vi "SummaryWithGlyphManager.vi"(8 "error in":errorcluster, 9 "glyph manager":T1, 10 "depth":i32, 11 "node self ref":T3) -> (0 "error out":errorcluster, 1 "glyph manager out":T1, 2 "summary":T4[](array[typedef]))   [LabVIEW 2025, in "CEF.lvlib"]
doc: "Gets the summary of a node and all the subnodes. This description can be used to update the tree controlCopyright 2017 National Instruments Corporation\n\nLicensed under the Apache License, Version 2.0 (the \"License\"); you may not use this file except in compliance with the License. You may obtain a copy of the License at http://www.apache.org/licenses/LICENSE-2.0\nUnless required by applicable law or agreed to in writing, software distributed under the License is distributed on an \"AS IS\" BASIS, WITHOUT WARRANTIES OR CONDITIONS OF ANY KIND, either express or implied. See the License for the specific language governing permissions and limitations under the License."
uses:
  CEF.lvlib
  Node/Summary.ctl
  Node/NodeRef.ctl
  Node/CEF_Node.lvclass
  glyph manager/glyph manager.ctl
  <vilib>/picture/picture.llb/imagedata.ctl
  Node/CEF_Node.lvclass/CEF_Node.ctl
  Node/ReadParent.vi
  Node/ReadChildren.vi
  Node/ReadNodeClass.vi
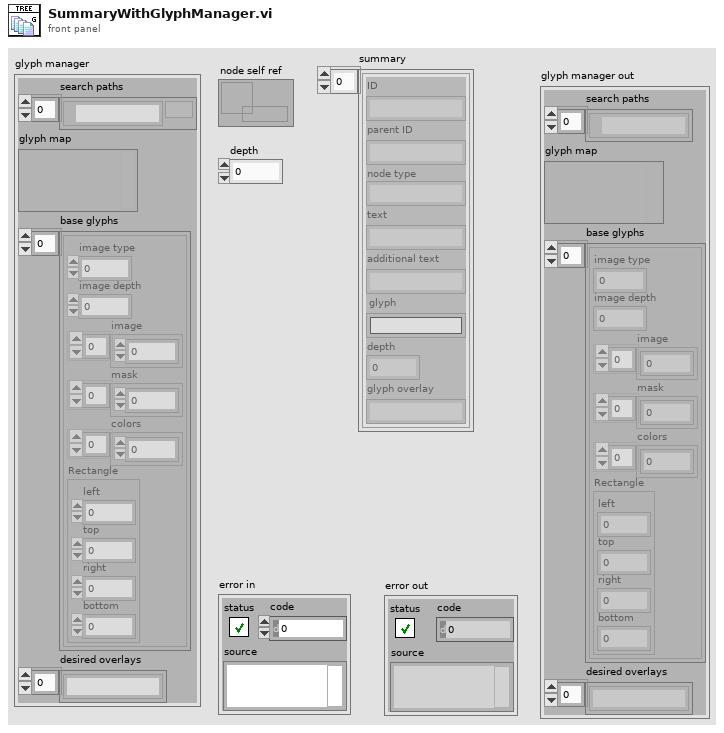
[diagram p1: front panel]
types:
  T1 = typedef "CEF.lvlib/glyph manager.ctl" = cluster{"search paths":path[], "glyph map":variant, "base glyphs":T2[], "desired overlays":string[]}
  T2 = typedef "imagedata.ctl" = cluster{"image type":i32, "image depth":i32, "image":u8[], "mask":u8[], "colors":u32[], "Rectangle":cluster{"left":i16, "top":i16, "right":i16, "bottom":i16}}
  T3 = typedef "CEF.lvlib/CEF_Node.lvclass/NodeRef.ctl" = refnum<data-value>
  T4 = typedef "CEF.lvlib/CEF_Node.lvclass/Summary.ctl" = cluster{"ID":string, "parent ID":string, "node type":string, "text":string, "additional text":string, "glyph":string, "depth":i32, "glyph overlay":string}
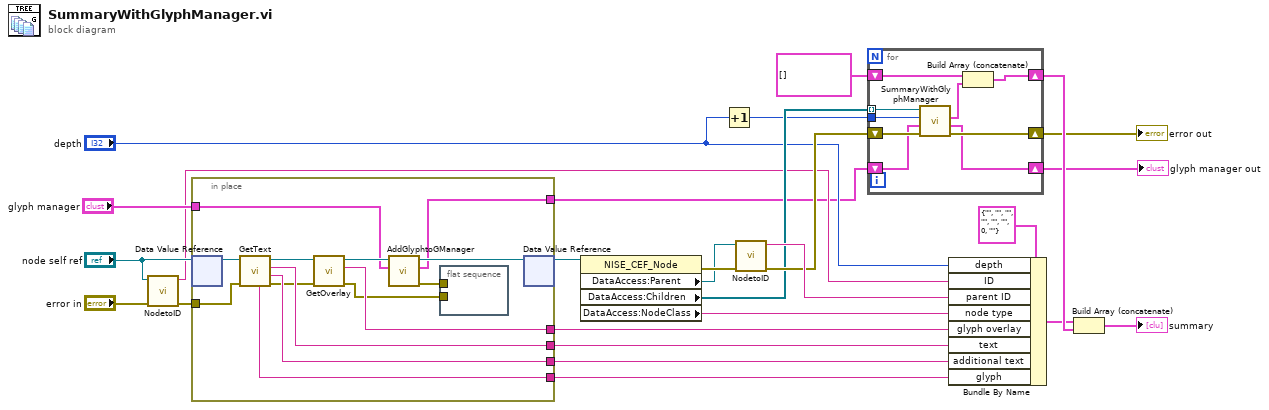
[diagram p0: block diagram]
diagram:
  n1 = call "NodetoID.vi"("error in"="error in", "node ref"="node self ref") -> ("error out"=w23:errorcluster, "ID"=w3:string)  [unwired: 8 in]
  n2 = in-place {
    in-place-border: [w40] -> w6
    in-place-border: [w39] -> w7
    in-place-border: [w38] -> w5
    in-place-border: w23 -> [w37]
    in-place-border: [w33] -> w8
    in-place-border: "glyph manager" -> [w28]
    in-place-border: [w27] -> w2
    n3 = in-place-dvr #1("node self ref") -> (w36:refnum<class "CEF_Node.lvclass">)  [unwired: 1 out]
    n4 = call-dynamic "GetText.vi"("error in"=w37, "CEF_Node in"=w36) -> ("error out"=w34:errorcluster, "additional text"=w40:string, "text"=w39:string, "CEF_Node out"=w35:refnum<class "CEF_Node.lvclass">, "glyph"=w38:string)  [unwired: 5 in]
    n5 = call-dynamic "GetOverlay.vi"("error in"=w34, "CEF_Node in"=w35) -> ("error out"=w29:errorcluster, "overlay"=w33:string, "CEF_Node out"=w32:refnum<class "CEF_Node.lvclass">)  [unwired: 7 in]
    n6 = call-dynamic "AddGlyphtoGManager.vi"("glyph manager"=w28, "CEF_Node in"=w32) -> ("error out"=w30:errorcluster, "glyph manager out"=w27:T1, "CEF_Node out"=w31:refnum<class "CEF_Node.lvclass">)  [unwired: 7 in]
    n7 = flat-sequence {
      tunnel: w30 -> [_]
      tunnel: w29 -> [_]
      frame #0 {
      }
    }
    n8 = in-place-dvr #1(w31) -> (w4:T3)  [unwired: 1 out]
  }
  n9 = property class="NISE_CEF_Node"(reference=w4) -> (error out=w19:errorcluster, "DataAccess:Parent"=w18:T3, "DataAccess:Children"=w17:T3[], "DataAccess:NodeClass"=w21:string)  [unwired: 1 in, 1 out]
  n10 = Increment(x="depth") -> (x+1=w13:i32)
  n11 = call "NodetoID.vi"("error in"=w19, "node ref"=w18) -> ("error out"=w20:errorcluster, "ID"=w22:string)  [unwired: 8 in]
  n12 = for {
    tunnel: w17 -> [w47] mode=indexing
    tunnel: w13 -> [w46]
    shift-right: [w48] -> w16
    shift-left: T4[] [] ("childrensummary") -> [w49]
    shift-right: [w44] -> w10
    shift-left: w20 -> [w45]
    shift-right: [w42] -> w1
    shift-left: w2 -> [w41]
    n13 = call "SummaryWithGlyphManager.vi"("error in"=w45, "glyph manager"=w41, "depth"=w46, "node self ref"=w47) -> ("error out"=w44:errorcluster, "glyph manager out"=w42:T1, "summary"=w43:T4[])  [unwired: 5 in]
    n14 = Build Array (concatenate)(w49, w43) -> (w48:T4[])
  }
  "error out" <- w10
  "glyph manager out" <- w1
  n15 = Bundle By Name(cluster=T4 {"ID"="", "parent ID"="", "node type"="", "text"="", "additional text"="", "glyph"="", "depth"=0, "glyph overlay"=""} ("nodeSummary"), "depth"="depth", "ID"=w3, "parent ID"=w22, "node type"=w21, "glyph overlay"=w8, "text"=w7, "additional text"=w6, "glyph"=w5) -> (w15:T4)
  n16 = Build Array (concatenate)(w15, w16) -> (→"summary":T4[])
